vi "InstaCoverage Time Measurement.vi"() -> (2 "ICov Results":enum16{"PASSED", "FAILED", "ERROR"}[](array[ring]), 3 "ICov Testing time (seconds)":dbl)   [LabVIEW 2018]
uses:
  <resource>/Framework/Providers/InstaCoverage/Pro/InstaCoverage_API/Run Tests From Project By Path.vi
  <resource>/Framework/Providers/InstaCoverage/Core/TestSuite/TestSuite.lvclass
  <resource>/Framework/Providers/InstaCoverage/Pro/InstaCoveragePro.lvlib
panel:
  out "Project Path":string
  # "ICov"
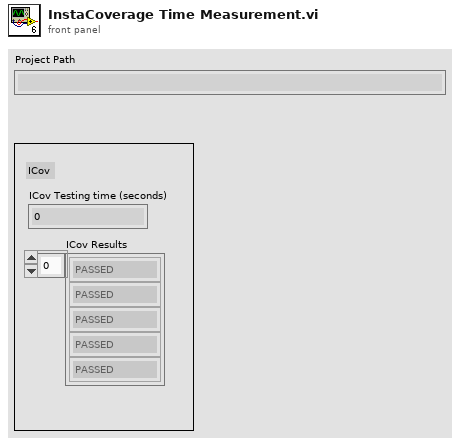
[diagram p1: front panel]
types:
  T1 = typedef "InstaCoverageCore.lvlib/APIResultEnum.ctl" = enum16{"PASSED", "FAILED", "ERROR", "NONE"}
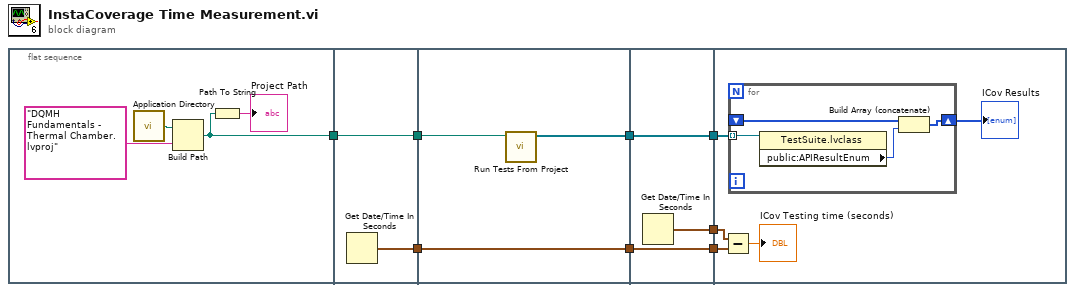
[diagram p0: block diagram]
diagram:
  n1 = flat-sequence {
    tunnel: [w10] -> w1
    tunnel: [w14] -> w5
    tunnel: [w13] -> w2
    tunnel: w1 -> [w13]
    tunnel: [w17] -> w6
    tunnel: w5 -> [w17]
    tunnel: [w16] -> w3
    tunnel: w2 -> [w15]
    tunnel: [w20] -> w8
    tunnel: [w19] -> w7
    tunnel: w6 -> [w19]
    tunnel: [w18] -> w4
    tunnel: w3 -> [w18]
    tunnel: w8 -> [w22]
    tunnel: w7 -> [w23]
    tunnel: w4 -> [w21]
    frame #0 {
      n2 = call <vilib>:"Application Directory.vi"() -> ("Application Directory"=w9:path)
      n3 = Build Path(base path=w9, name or relative path="DQMH Fundamentals - Thermal Chamber.lvproj") -> (appended path=w10:path)
      n4 = Path To String(path=w10) -> (string=→"Project Path":string)
    }
    frame #1 {
      n5 = Get Date/Time In Seconds() -> (seconds since 1Jan1904=w14:timestamp)
    }
    frame #2 {
      n6 = call-poly <resource>:"Run Tests From Project.vi"("Path lvProject"=w15) -> ("TestSuite[] results"=w16:refnum<class "TestSuite.lvclass">[])  [unwired: 9 in, 1 out]
    }
    frame #3 {
      n7 = Get Date/Time In Seconds() -> (seconds since 1Jan1904=w20:timestamp)
    }
    frame #4 {
      n8 = Subtract(x=w22, y=w23) -> (x-y=→"ICov Testing time (seconds)":dbl)
      n9 = for {
        shift-right: [w27] -> w25
        shift-left: _ -> [w28]
        tunnel: w21 -> [w26] mode=indexing
        n10 = property class="TestSuite.lvclass"(reference=w26) -> ("public:APIResultEnum"=w29:T1)  [unwired: 1 in, 2 out]
        n11 = Build Array (concatenate)(w28, w29) -> (w27:T1[])
      }
      "ICov Results" <- w25
    }
  }
